vi "Read 1D Barcode.vi"() -> ()   [LabVIEW 2018]
doc: "This example shows how to use the IMAQ Read Barcode VI to locate and read standard 1D barcodes."
uses:
  <vilib>/vision/Instrument.llb/Barcode Search Options.ctl
  <vilib>/vision/NI_Vision_Development_Module.lvlib
panel:
  out "Barcode ANSI/CEN/ISO Grading Report":T1(array[cluster])
  out "Barcode Read":cluster{"Data":string, "Barcode Type":string}[](array[cluster])
  out "Number of Barcodes Found":u32
  out "Image":T2(plugin-control)
  in  "Delay (s.)":dbl(slide)=0.4897959183673469 scale=0.0..2.0
  in  "Stop":bool
  # "Overview: Demonstrate the use of the Read Barcode 2 function of Vision Development Module.\nRequirements: Vision Development Module\nInstructions: Run the VI."
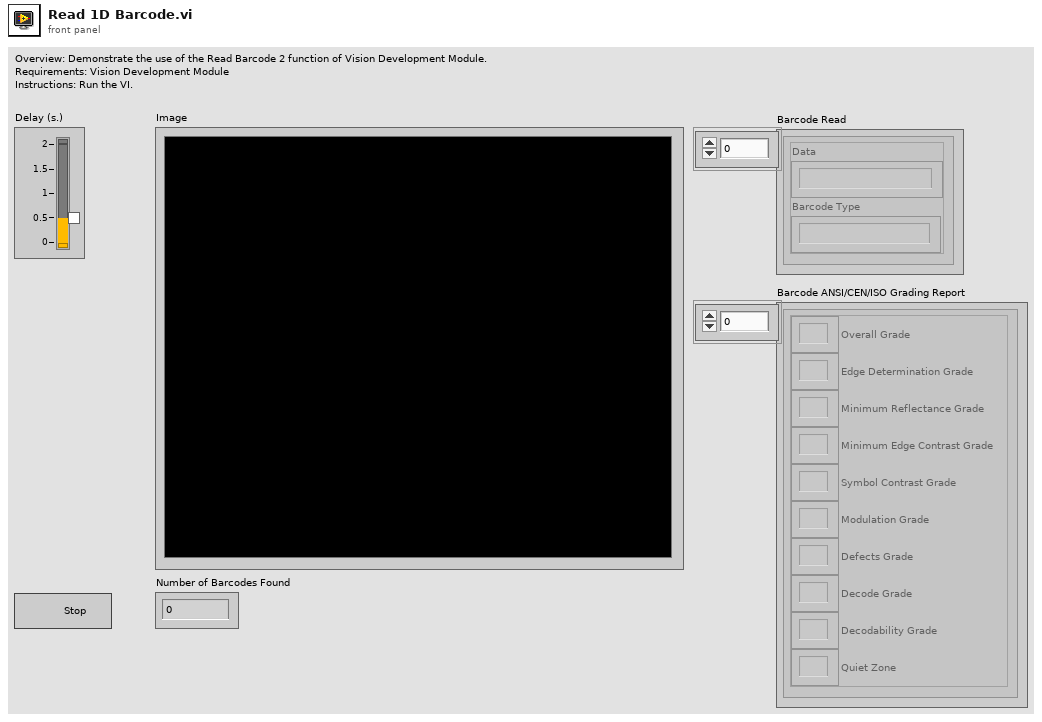
[diagram p1: front panel]
types:
  T1 = cluster{"Overall Grade":string, "Edge Determination Grade":string, "Minimum Reflectance Grade":string, "Minimum Edge Contrast Grade":string, "Symbol Contrast Grade":string, "Modulation Grade":string, "Defects Grade":string, "Decode Grade":string, "Decodability Grade":string, "Quiet Zone":string}[]
  T2 = typedef "IMAQ Image.ctl" = refnum<image>
  T3 = cluster{"Calculate Grading Report":bool, "Scan Width ":i32}
  T4 = typedef "Barcode Search Options.ctl" = cluster{"Min Bar Width":u32, "Min Edge Strength":u32, "Min Bars":u32, "Skip Location Search?":bool}
  T5 = cluster{"Data":string, "Special Char 1":string, "Special Char 2":string, "Checksum(s)":string, "Barcode Type":u32, "Confidence Level":sgl, "Bounding Box":cluster{"x":sgl, "y":sgl}[]}[]
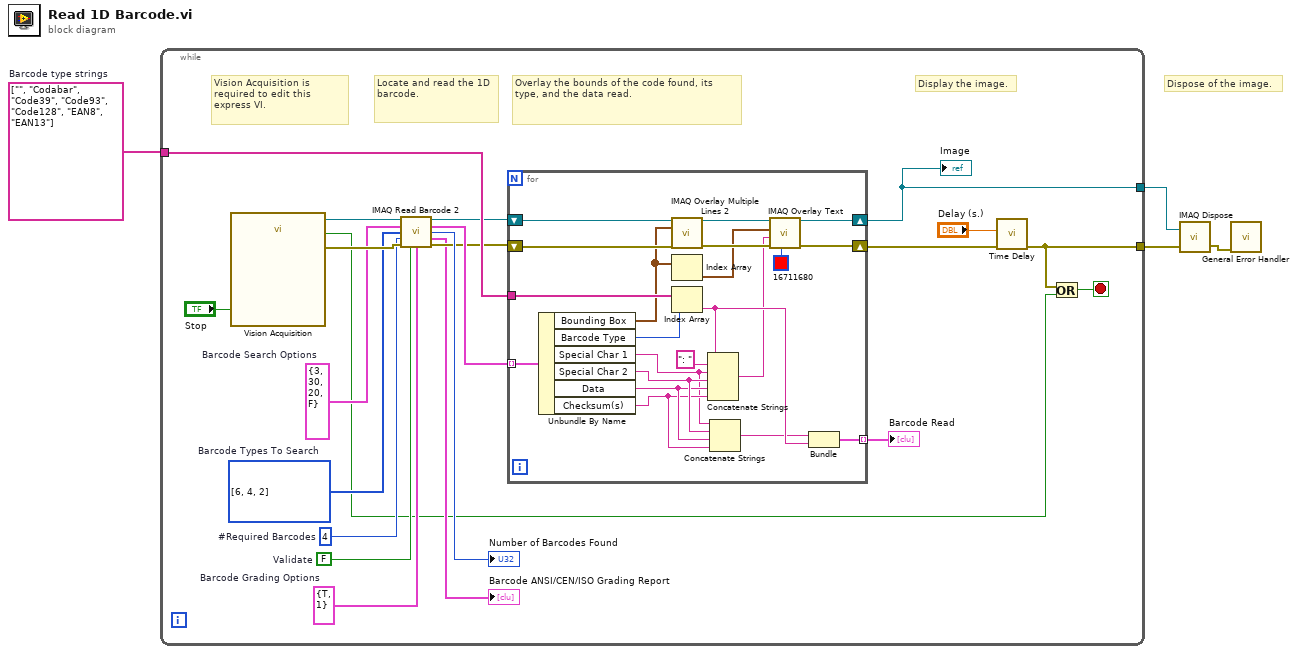
[diagram p0: block diagram]
diagram:
  w3 = string[] ["", "Codabar", "Code39", "Code93", "Code128", "EAN8", "EAN13"]  # Barcode type strings
  # "Dispose of the image."
  n1 = while {
    tunnel: [w12] -> w4
    tunnel: [w6] -> w2
    tunnel: w3 -> [w20]
    stop <- w25 stop-if-true
    w9 = T3 {"Calculate Grading Report"=TRUE, "Scan Width "=1}  # Barcode Grading Options
    w10 = T4 {"Min Bar Width"=3, "Min Edge Strength"=30, "Min Bars"=20, "Skip Location Search?"=FALSE}  # Barcode Search Options
    w22 = u32 4  # #Required Barcodes
    w16 = u32[] [6, 4, 2] items=["Reserved", "Codabar", "Code 39", "Code 93", "Code 128", "EAN 8", "EAN 13", "Interleaved 2 of 5", "MSI", "UPCA", "Pharmacode", "RSS Limited"]  # Barcode Types To Search
    w11 = FALSE  # Validate
    # "Display the image."
    # "Locate and read the 1D barcode."
    # "Vision Acquisition is required to edit this express VI."
    # "Overlay the bounds of the code found, its type, and the data read."
    n2 = call "Vision Acquisition"("Stop (F)"="Stop") -> ("Image Out"=w18:T2, "Stopped"=w5:bool, "error out"=w23:errorcluster)  [unwired: 24 in]
    n3 = call "IMAQ Read Barcode 2"("Image"=w18, "Barcode Search Options"=w10, "Barcode Types To Search"=w16, "Num of Required Barcodes"=w22, "error in (no error)"=w23, "Validate"=w11, "Barcode Grading Options"=w9) -> ("Image (duplicate)"=w19:T2, "Barcodes"=w21:T5, "Num of Barcodes"=→"Number of Barcodes Found":u32, "Barcode ANSI/CEN/ISO Grading Report"=→"Barcode ANSI/CEN/ISO Grading Report":T1, "error out"=w15:errorcluster)  [unwired: 4 in]
    n4 = for {
      tunnel: w21 -> [w46] mode=indexing
      tunnel: w20 -> [w45]
      shift-right: [w41] -> w12
      shift-left: w19 -> [w37]
      shift-right: [w38] -> w14
      shift-left: w15 -> [w40]
      tunnel: [w33] -> w8 mode=indexing
      n5 = Unbundle By Name(w46) -> ("Bounding Box"=w36:cluster{"x":sgl, "y":sgl}[], "Barcode Type"=w34:u32, "Special Char 1"=w26:string, "Special Char 2"=w30:string, "Data"=w29:string, "Checksum(s)"=w28:string)
      n6 = call "IMAQ Overlay Multiple Lines 2"("Image"=w37, "Line End Points"=w36, "error in (no error)"=w40) -> ("Image Out"=w43:T2, "error out"=w39:errorcluster)  [unwired: 11 in]
      n7 = Index Array(array=w36) -> (element=w35:cluster{"x":sgl, "y":sgl})  [unwired: 1 in]
      n8 = Index Array(array=w45, index=w34) -> (element=w32:string)
      n9 = Concatenate Strings(w32, ": " ("string"), w26, w30, w29, w28) -> (w31:string)
      n10 = Concatenate Strings(w26, w30, w29, w28) -> (w27:string)
      n11 = call "IMAQ Overlay Text"("Text Color (black)"=u32 16711680, "error in (no error)"=w39, "String"=w31, "Origin"=w35, "Image"=w43) -> ("error out"=w38:errorcluster, "Image Out"=w41:T2)  [unwired: 5 in]
      n12 = Bundle(w27, w32) -> (w33:cluster{string, string})  [unwired: 1 in]
    }
    "Image" <- w12
    "Barcode Read" <- w8
    n13 = call "Time Delay"("error in (no error)"=w14, "Delay Time (s)"="Delay (s.)") -> ("error out"=w6:errorcluster)  [unwired: 9 in]
    n14 = Or(x=w6, y=w5) -> (x .or. y?=w25:bool)
  }
  n15 = call "IMAQ Dispose"("Image"=w4, "error in (no error)"=w2) -> ("error out"=w1:errorcluster)  [unwired: 1 in, 3 out]
  n16 = call <vilib>:"General Error Handler.vi"("error in (no error)"=w1) -> ()  [unwired: 10 in, 5 out]
